vi "Resize.vi"(4 "Send events? [T]":bool=TRUE, 6 "Defer Panel Updates? [T]":bool=TRUE, 7 "VI Refnum":refnum<vi>, 8 "error in (no error)":errorcluster, 10 "Bounds":T1, 11 "MMI Scaling in":refnum<class "IObject.lvclass">) -> (0 "error out":errorcluster, 2 "Resized":string[](array[string]), 3 "MMI Scaling out":refnum<class "IObject.lvclass">)   [LabVIEW 2013, in "IObject.lvclass"]
uses:
  IObject.lvclass
  <vilib>/Utility/miscctls.llb/LVRectTypeDef.ctl
  IObject.lvclass/IObject.ctl
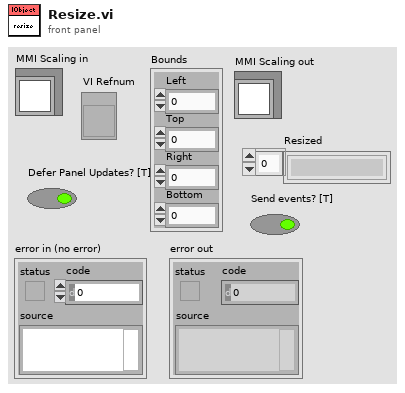
[diagram p1: front panel]
types:
  T1 = typedef "LVRectTypeDef.ctl" = cluster{"Left":i16, "Top":i16, "Right":i16, "Bottom":i16}
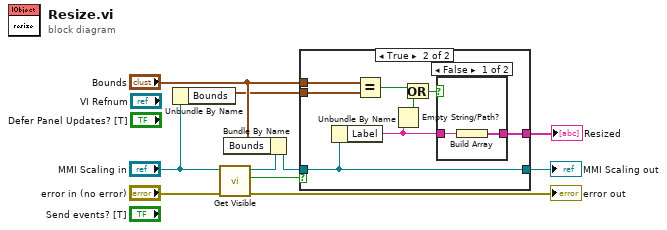
[diagram p0: block diagram]
diagram:
  n1 = Unbundle By Name("MMI Scaling in") -> ("Bounds"=w1:T1)
  n2 = call-dynamic "Get Visible.vi"("error in (no error)"="error in (no error)", "IObject in"="MMI Scaling in") -> ("error out"=→"error out":errorcluster, "Visible?"=w6:bool, "IObject out"=w4:refnum<class "IObject.lvclass">)  [unwired: 6 in, 1 out]
  n3 = Bundle By Name(cluster=w4, "Bounds"="Bounds") -> (w3:refnum<class "IObject.lvclass">)
  n4 = case shown="True" w6 {
    tunnel: [_ w16] -> w9
    tunnel: "Bounds" -> [_ w15]
    tunnel: w3 -> [w11 w14]
    tunnel: [w11 w14] -> w5
    tunnel: w1 -> [_ w12]
    frame False {
    }
    frame True {
      n5 = Unbundle By Name(w14) -> ("Label"=w13:string)
      n6 = Equal?(x=w15, y=w12) -> (x = y?=w19:bool)
      n7 = Empty String/Path?(string/path=w13) -> (empty?=w18:bool)
      n8 = Or(x=w19, y=w18) -> (x .or. y?=w17:bool)
      n9 = case shown="False" w17 {
        tunnel: [w21 _] -> w16
        tunnel: w13 -> [w20 _]
        frame False {
          n10 = Build Array(w20) -> (w21:string[])
        }
        frame True {
        }
      }
    }
  }
  "MMI Scaling out" <- w5
  "Resized" <- w9
